vi "get channels test.vi"() -> ()   [LabVIEW 2014, in "OPC UA Client Tests.lvlib"]
uses:
  OPC UA Client Tests.lvlib
  module/configuration/OPC UA Client configuration.lvclass
panel:
  out "error out":errorcluster
  out "channels match":bool
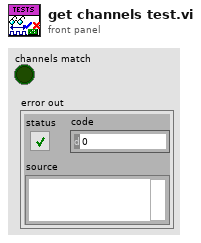
[diagram p1: front panel]
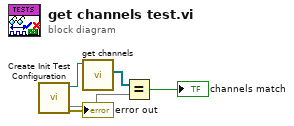
[diagram p0: block diagram]
diagram:
  n1 = call "Create Init Test Configuration.vi"() -> ("error out"=→"error out":errorcluster, "module"=w3:refnum<class "OPC UA Client configuration.lvclass">, 4:w1)  [unwired: 8 in, 1 out]
  n2 = call-dynamic "get channels.vi"("OPC UA configuration in"=w3) -> ("channels"=w5:refnum<class "TBM channel.lvclass">[])  [unwired: 9 in, 1 out]
  n3 = Equal?(x=w5, y=w1) -> (x = y?=→"channels match":bool)
